vi "Init Instruments.vi"(8 "error in (no error)":errorcluster, 11 "Host MSS Test Actor in":refnum<class "Host MSS Test Actor.lvclass">) -> (0 "error out":errorcluster, 3 "Host MSS Test Actor out":refnum<class "Host MSS Test Actor.lvclass">)   [LabVIEW 2023]
uses:
  <vilib>/Utility/error.llb/Error Cluster From Error Code.vi
  <vilib>/ErrorRing/Error Ring.xnode
  Host MSS Test Actor.lvclass
  C:/Program Files/National Instruments/LabVIEW 2023/vi.lib/ActorFramework/Actor/Actor.lvclass
  D:/git/HAL/HAL GOOP4/Host Measure and Stimulus Subsystems/Tests/Host MSS Test Actor/Host MSS Test Actor/Host MSS Test Actor.lvclass
  C:/Program Files/National Instruments/LabVIEW 2023/vi.lib/ni/Actors/Network Endpoint Actors/Nested Endpoint Caller/Nested Endpoint Caller/Nested Endpoint Caller.lvclass
  <vilib>/ActorFramework/Message Enqueuer/Message Enqueuer.lvclass
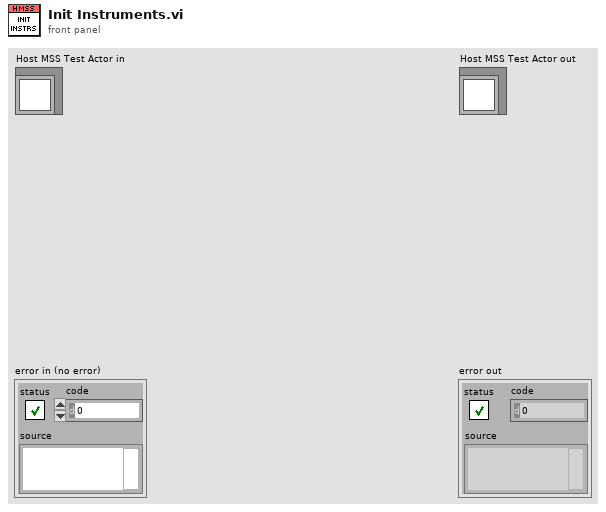
[diagram p1: front panel]
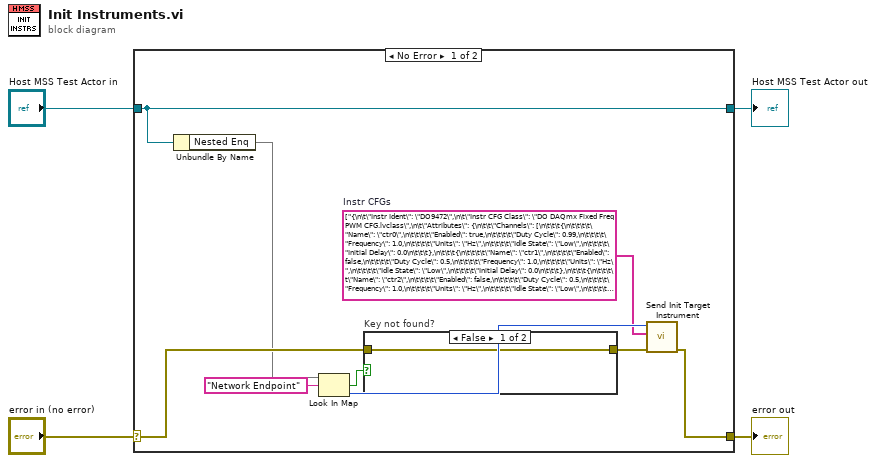
[diagram p0: block diagram]
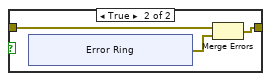
[diagram p2: hidden frame]
diagram:
  n1 = case shown="No Error" "error in (no error)" {
    selector: "error in (no error)" -> [w7 w24]
    tunnel: [w6 w24] -> w3
    tunnel: [w8 w23] -> w1
    tunnel: "Host MSS Test Actor in" -> [w8 w23]
    frame No Error {
      w11 = string[] ["{\n\t\"Instr Ident\": \"DO9472\",\n\t\"Instr CFG Class\": \"DO DAQmx Fixed Freq PWM CFG.lvclass\",\n\t\"Attributes\": {\n\t\t\"Channels\": [\n\t\t\t{\n\t\t\t\t\"Name\": \"ctr0\",\n\t\t\t\t\"Enabled\": true,\n\t\t\t\t\"Duty Cycle\": 0.99,\n\t\t\t\t\"Frequency\": 1.0,\n\t\t\t\t\"Units\": \"Hz\",\n\t\t\t\t\"Idle State\": \"Low\",\n\t\t\t\t\"Initial Delay\": 0.0\n\t\t\t},\n\t\t\t{\n\t\t\t\t\"Name\": \"ctr1\",\n\t\t\t\t\"Enabled\": false,\n\t\t\t\t\"Duty Cycle\": 0.5,\n\t\t\t\t\"Frequency\": 1.0,\n\t\t\t\t\"Units\": \"Hz\",\n\t\t\t\t\"Idle State\": \"Low\",\n\t\t\t\t\"Initial Delay\": 0.0\n\t\t\t},\n\t\t\t{\n\t\t\t\t\"Name\": \"ctr2\",\n\t\t\t\t\"Enabled\": false,\n\t\t\t\t\"Duty Cycle\": 0.5,\n\t\t\t\t\"Frequency\": 1.0,\n\t\t\t\t\"Units\": \"Hz\",\n\t\t\t\t\"Idle State\": \"Low\",\n\t\t\t\t\"Initial Delay\": 0.0\n\t\t\t},\n\t\t\t{\n\t\t\t\t\"Name\": \"ctr3\",\n\t\t\t\t\"Enabled\": false,\n\t\t\t\t\"Duty Cycle\": 0.5,\n\t\t\t\t\"Frequency\": 1.0,\n\t\t\t\t\"Units\": \"Hz\",\n\t\t\t\t\"Idle State\": \"Low\",\n\t\t\t\t\"Initial Delay\": 0.0\n\t\t\t}\n\t\t],\n\t\t\"Timing\": {\n\t\t\t\"Samples per Channel\": 1000,\n\t\t\t\"Sample Mode\": \"Continuous Samples\",\n\t\t\t\"Sample Rate\": 0.0,\n\t\t\t\"Sample Clock Source\": \"Implicit\",\n\t\t\t\"Active Edge\": \"Rising\"\n\t\t},\n\t\t\"Trigger\": {\n\t\t\t\"Trigger Type\": \"No Trigger\"\n\t\t}\n\t}\n}", "{\n    \"Instr Ident\": \"TC9210\",\n    \"Instr CFG Class\": \"Thermometer DAQmx Base CFG.lvclass\",\n    \"Attributes\": {\n        \"Channels\": [\n            {\n                \"Name\": \"ai0\",\n                \"Enabled\": true,\n                \"CJC Source\": \"Constant Value\",\n                \"Max Degree\": 100,\n                \"Min Degree\": 0,\n                \"CJC Value\": 25,\n                \"Thermocouple Type\": \"J\",\n                \"Units\": \"Deg C\",\n                \"CJC Channel\": \"\",\n                \"Enable Autozero\": false,\n                \"Autozero Mode\": \"None\"\n            },\n            {\n                \"Name\": \"ai1\",\n                \"Enabled\": false,\n                \"CJC Source\": \"Constant Value\",\n                \"Max Degree\": 100,\n                \"Min Degree\": 0,\n                \"CJC Value\": 25,\n                \"Thermocouple Type\": \"J\",\n                \"Units\": \"Deg C\",\n                \"CJC Channel\": \"\",\n                \"Enable Autozero\": false,\n                \"Autozero Mode\": \"None\"\n            },\n            {\n                \"Name\": \"ai2\",\n                \"Enabled\": false,\n                \"CJC Source\": \"Constant Value\",\n                \"Max Degree\": 100,\n                \"Min Degree\": 0,\n                \"CJC Value\": 25,\n                \"Thermocouple Type\": \"J\",\n                \"Units\": \"Deg C\",\n                \"CJC Channel\": \"\",\n                \"Enable Autozero\": false,\n                \"Autozero Mode\": \"None\"\n            },\n            {\n                \"Name\": \"ai3\",\n                \"Enabled\": false,\n                \"CJC Source\": \"Constant Value\",\n                \"Max Degree\": 100,\n                \"Min Degree\": 0,\n                \"CJC Value\": 25,\n                \"Thermocouple Type\": \"J\",\n                \"Units\": \"Deg C\",\n                \"CJC Channel\": \"\",\n                \"Enable Autozero\": false,\n                \"Autozero Mode\": \"None\"\n            }\n        ],\n        \"Timing\": {\n            \"Samples per Channel\": 1000,\n            \"Sample Mode\": \"Continuous Samples\",\n            \"Sample Rate\": 14,\n            \"Sample Clock Source\": \"OnboardClock\",\n            \"Active Edge\": \"Rising\"\n        },\n        \"Trigger\": {\n            \"Trigger Type\": \"No Trigger\"\n        },\n        \"Acquisition\": {\n            \"Relative To\": \"Current Read Position\",\n            \"Overwrite\": \"Do Not Overwrite Unread Samples\",\n            \"Samples per Fetch\": -1,\n            \"Timeout\": 1\n        }\n    }\n}"]  # Instr CFGs
      n2 = Unbundle By Name(w8) -> ("Nested Enq"=w5)
      n3 = Look In Map(map=w5, key="Network Endpoint") -> (key not found?=w10:bool, value=w12:i32)  [unwired: 1 in]
      n4 = case "Key not found?" shown="False" w10 {
        tunnel: w7 -> [w14 w17]
        tunnel: [w14 w16] -> w9
        frame False {
        }
        frame True {
          n5 = xnode "Error Ring"() -> ("error out"=w15:errorcluster)
          n6 = Merge Errors(w17, w15) -> (w16:errorcluster)
        }
      }
      n7 = call "Send Init Target Instrument.vi"("error in (no error)"=w9, "Physical Instr CFGs"=w11, "Message Enqueuer"=w12) -> ("error out"=w6:errorcluster)  [unwired: 7 in, 1 out]
    }
    frame Error {
    }
  }
  "error out" <- w3
  "Host MSS Test Actor out" <- w1
